vi "Bertta_v06_2.vi"() -> ()   [LabVIEW 2015]
uses:
  x64/Debug/BERTTA.dll
panel:
  in  "s":bool
  out "Numeric 4":dbl
  in  "Tab Control":T1(tab)
  in  "Description":string
  in  "Project name":string
  in  "User (initials)":string
  out "Tr":dbl
  out "Tj":dbl
  out "Numeric 2":dbl
  out "Numeric 3":dbl
  out "Numeric":dbl
  out "Mettler 5":dynamicdata(graph)
  out "Temp":dynamicdata(graph)
  out "Mettler":dynamicdata(graph)
  in  "Balances":bool[](array[boolean])
  out "Waveform Chart 3":dynamicdata(graph)
  out "Table":string[][](table)
  in  "Headers":string[](array[string])
  in  "?":bool
  in  "Seq":dbl[][](array[numeric])=[[20.0, 40.0, 50.0], [40.0, 50.0, 20.0], [3.0, 3.0, 3.0]]
  out "Sp":dbl
  out "T":dbl
  out "Tinit":dbl
  out "Tset":dbl
  out "Time limit":dbl
  out "Step":i32
  out "Waveform Chart":dynamicdata(graph)
  in  "Tbypass":dbl=20.0
  in  "Tfail":dbl=22.0
  in  "err":i32
  in  "PAUSE":bool
  out "Tj in":dbl
  out "Tj out":dbl
  out "DT":dbl
  out "Elapsed":i32 format="%<%H:%M:%S>t"
  out "Waveform Chart 2":dynamicdata(graph)
  out "Rate (g/s)":dbl
  out "Time (s)":dbl
  out "Target (g)":dbl
  in  "Seq 2":dbl[][](array[numeric])=[[20.0, 60.0, 40.0], [60.0, 40.0, 20.0], [100.0, 100.0, 100.0]]
  out "Weight (1)":dbl
  out "target reached":i32
  out "x/y":dbl
  out "bal_previous":i32
  out "Step":i32
  in  "?":bool
  in  "Bypass ramp":dbl
  in  "bypass 2":bool
  out "DAQ assistant (4-20 mA)":dbl
  out "Step":i32
  out "bal_previous":i32
  out "x/y":dbl
  out "target reached":i32
  out "Waveform Chart 5":dynamicdata(graph)
  out "Weight (2)":dbl
  out "Rate (g/s)":dbl
  out "Time (s)":dbl
  out "Target (g)":dbl
  in  "Seq 3":dbl[][](array[numeric])=[[20.0, 60.0, 40.0], [60.0, 40.0, 20.0], [100.0, 100.0, 100.0]]
  in  "Boolean":bool
  in  "Bypass ramp":dbl
  in  "bypass":bool
  out "RS232 to Ismatec":dbl
  in  "Boolean 2":bool
  out "Step":i32
  out "bal_previous":i32
  out "x/y":dbl
  out "target reached":i32
  out "Waveform Chart 6":dynamicdata(graph)
  out "Weight (3)":dbl
  out "Rate (g/s)":dbl
  out "Time (s)":dbl
  out "Target (g)":dbl
  in  "Seq 4":dbl[][](array[numeric])=[[20.0, 60.0, 40.0], [60.0, 40.0, 20.0], [100.0, 100.0, 100.0]]
  in  "Boolean 3":bool
  out "Step":i32
  out "bal_previous":i32
  out "x/y":dbl
  out "target reached":i32
  out "Waveform Chart 7":dynamicdata(graph)
  out "Weight (4)":dbl
  out "Rate (g/s)":dbl
  out "Time (s)":dbl
  out "Target (g)":dbl
  in  "Seq 5":dbl[][](array[numeric])=[[20.0, 60.0, 40.0], [60.0, 40.0, 20.0], [100.0, 100.0, 100.0]]
  out "RPM":dbl
  out "Torque":dbl
  in  "Set RPM":dbl(slide) scale=0.0..500.0
  out "Waveform Chart 4":dynamicdata(graph)
  in  "?":T2(tab)
  in  "Device port":dbl=9.0
  out "Debug msg":dbl
  in  "Device port":dbl=13.0
  in  "Device port":i32=10
  in  "Device port 2":i32=11
  in  "Device port 3":i32=12
  in  "Device port 4":i32=15
  # "1"
  # "2"
  # "3"
  # "4"
  # "Step 1"
  # "Step 2"
  # "Step 3"
  # "Step 4"
  # "Step 1"
  # "Step 2"
  # "Step 3"
  # "Step 4"
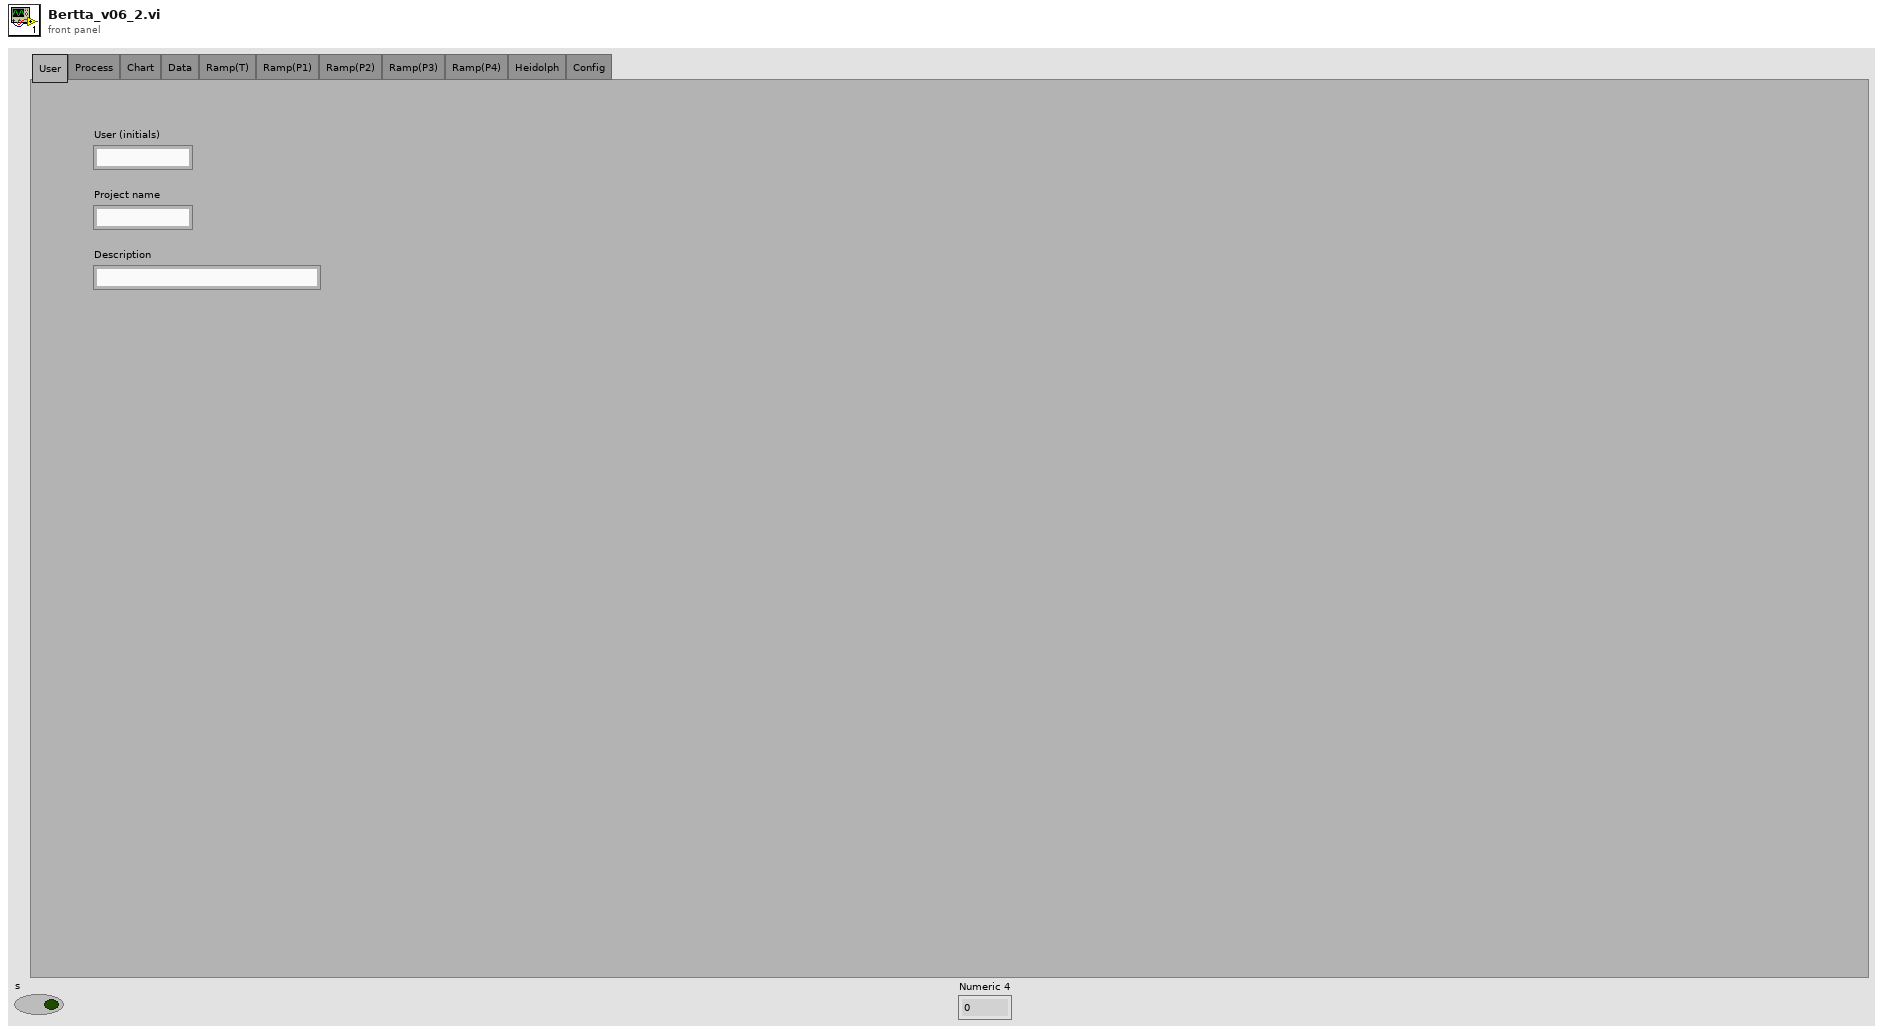
[diagram p1: front panel]
types:
  T1 = enum32{"User", "Process", "Chart", "Data", "Ramp(T)", "Ramp(P1)", "Ramp(P2)", "Ramp(P3)", "Ramp(P4)", "Heidolph", "Config"}
  T2 = enum32{"DB / File", "Lauda", "Heidolph", "Mettler 1", "Mettler 2", "Mettler 3", "Ismatec 1"}
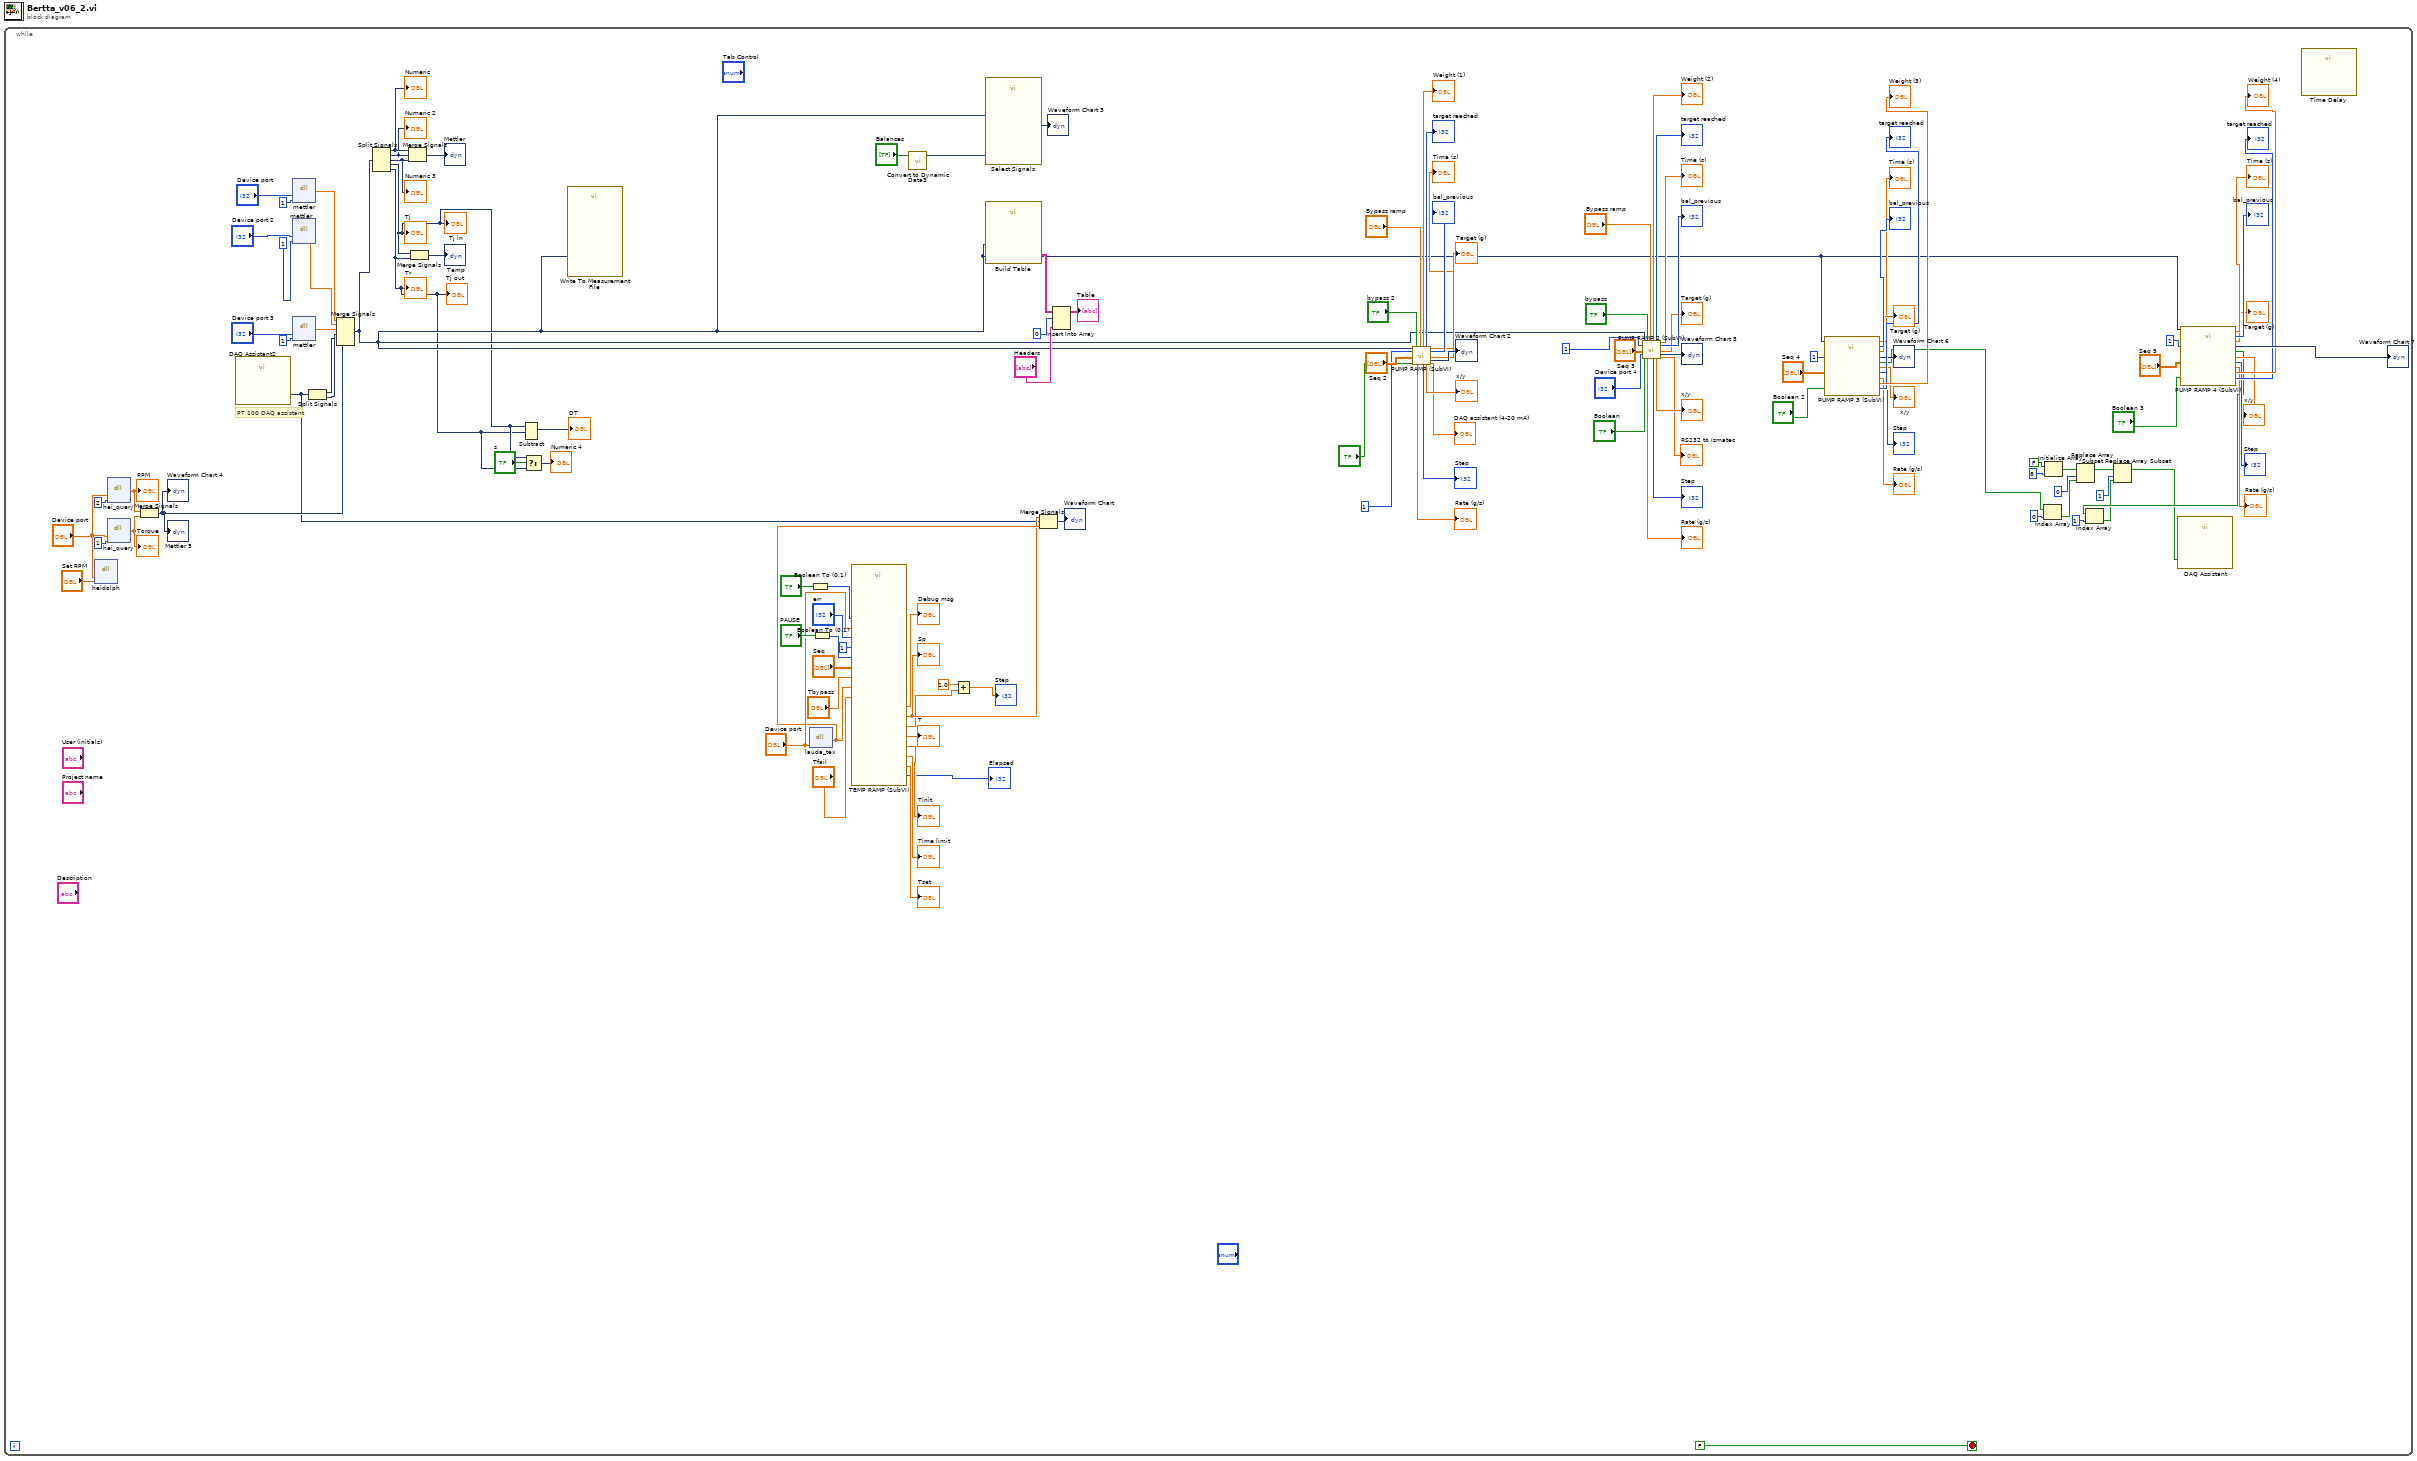
[diagram p0: block diagram]
diagram:
  n1 = while {
    stop <- FALSE stop-if-true
    # "PT 100 DAQ assistant"
    n2 = dll-call lib="C:/Users/shresplab/OneDrive - Kemira Oyj/Documents/Visual Studio 2017/Projects/Bertta/BERTTA/x64/Debug/BERTTA.dll" fn="heidolph"("port"="Device port", "speed"="Set RPM") -> ()  [unwired: 6 in, 2 out]
    n3 = dll-call lib="C:/Users/shresplab/OneDrive - Kemira Oyj/Documents/Visual Studio 2017/Projects/Bertta/BERTTA/x64/Debug/BERTTA.dll" fn="hei_query"("port"="Device port", "q"=2) -> ("return type"=w113:dbl)  [unwired: 5 in, 2 out]
    "RPM" <- w113
    n4 = dll-call lib="C:/Users/shresplab/OneDrive - Kemira Oyj/Documents/Visual Studio 2017/Projects/Bertta/BERTTA/x64/Debug/BERTTA.dll" fn="hei_query"("port"="Device port", "q"=1) -> ("return type"=w112:dbl)  [unwired: 5 in, 2 out]
    "Torque" <- w112
    n5 = Merge Signals(w113, w112) -> (w19:dynamicdata)
    "Waveform Chart 4" <- w19
    "Mettler 5" <- w19
    n6 = call "DAQ Assistant2"() -> ("data"=w4:dynamicdata)  [unwired: 17 in, 2 out]
    n7 = dll-call lib="C:/Users/shresplab/OneDrive - Kemira Oyj/Documents/Visual Studio 2017/Projects/Bertta/BERTTA/x64/Debug/BERTTA.dll" fn="mettler"("port"="Device port", "msg"=1) -> ("return type"=w85:dbl)  [unwired: 5 in, 2 out]
    n8 = dll-call lib="C:/Users/shresplab/OneDrive - Kemira Oyj/Documents/Visual Studio 2017/Projects/Bertta/BERTTA/x64/Debug/BERTTA.dll" fn="mettler"("port"="Device port 2", "msg"=1) -> ("return type"=w84:dbl)  [unwired: 5 in, 2 out]
    n9 = dll-call lib="C:/Users/shresplab/OneDrive - Kemira Oyj/Documents/Visual Studio 2017/Projects/Bertta/BERTTA/x64/Debug/BERTTA.dll" fn="mettler"("port"="Device port 3", "msg"=1) -> ("return type"=w71:dbl)  [unwired: 5 in, 2 out]
    n10 = Split Signals(w4) -> (w10:dynamicdata, w51:dynamicdata)  [unwired: 2 in]
    n11 = Merge Signals(w85, w84, w71, w51, w10, w19) -> (w17:dynamicdata)
    n12 = Split Signals(w17) -> (w24:dynamicdata, w22:dynamicdata, w21:dynamicdata, w16:dynamicdata, w15:dynamicdata)  [unwired: 5 in]
    "Numeric" <- w24
    "Numeric 2" <- w22
    "Numeric 3" <- w21
    "Tr" <- w15
    "Tj" <- w16
    "Tj in" <- w16
    "Tj out" <- w15
    n13 = Merge Signals(w24, w22, w21) -> (→"Mettler":dynamicdata)
    n14 = Merge Signals(w16, w15) -> (→"Temp":dynamicdata)
    n15 = Subtract(1:w15, 2:w16) -> (0:→"DT":dynamicdata)  [unwired: 1 in, 1 out]
    n16 = Select(t=w16, s="s", f=w15) -> (s? t:f=→"Numeric 4":dynamicdata)
    n17 = call "Write To Measurement File"("Signals"=w17) -> ()  [unwired: 16 in, 3 out]
    n18 = dll-call lib="C:/Users/shresplab/OneDrive - Kemira Oyj/Documents/Visual Studio 2017/Projects/Bertta/BERTTA/x64/Debug/BERTTA.dll" fn="lauda_tex"("port"="Device port") -> ("return type"=w11:dbl)  [unwired: 4 in, 2 out]
    n19 = Boolean To (0,1)(Boolean="?") -> (0, 1=w66:i16)
    n20 = Boolean To (0,1)(Boolean="PAUSE") -> (0, 1=w20:i16)
    n21 = call "TEMP RAMP (SubVI).vi"("Device port"="Device port", "enable"=i16 1 ("Numeric"), "Tbyp"="Tbypass", "pause"=w20, "Seq"="Seq", "Tcurrent"=w11, "bypass"=w66, "err"="err", "Tfail"="Tfail") -> ("Step out"=w3:dbl, "T"=→"T":dbl, "Sp"=w7:dbl, "elapsed"=→"Elapsed":i32, "tr"=→"Time limit":dbl, "Debug msg"=→"Debug msg":dbl, "Tset"=→"Tset":dbl, "Tinit"=→"Tinit":dbl)  [unwired: 3 in]
    "Sp" <- w7
    n22 = call "Convert to Dynamic Data3"("Array"="Balances") -> ("Dynamic Data Type"=w119:dynamicdata)  [unwired: 3 in]
    n23 = Add(x=1.0, y=w3) -> (x+y=→"Step":dbl)
    n24 = call "Select Signals"("Selector Input"=w119, "Signals"=w17) -> ("Signal Out"=→"Waveform Chart 3":dynamicdata)  [unwired: 8 in, 1 out]
    n25 = call "Build Table"("Signals"=w17) -> ("Table"=w122:string[][])  [unwired: 4 in, 6 out]
    n26 = Merge Signals(w7, w4, w11) -> (→"Waveform Chart":dynamicdata)
    n27 = Insert Into Array(array=w122, index (row)=0, new element="Headers") -> (→"Table":string[][])  [unwired: 1 in]
    n28 = call "PUMP RAMP (SubVI).vi"("Dynamic Data"=w17, "Numeric"=i16 1, "Seq in"="Seq 2", 5:"?", "bypass"="bypass 2", "bypass RPM"="Bypass ramp") -> ("Rate (g/s)"=→"Rate (g/s)":dbl, "Weight (S1)"=→"Weight (1)":dbl, "Step 2"=→"Step":i32, "target reached"=→"target reached":i32, "x/y"=→"x/y":dbl, "Time (s)"=→"Time (s)":dbl, "bal_previous"=→"bal_previous":i32, "Target (g)"=→"Target (g)":dbl, "Waveform Chart 2"=→"Waveform Chart 2":dynamicdata, "DAQ assistant (4-20 mA)"=→"DAQ assistant (4-20 mA)":dbl)  [unwired: 4 in]
    n29 = call "PUMP RAMP 2 (SubVI).vi"("Dynamic Data"=w17, "Numeric"=i16 1, "Seq in"="Seq 3", "Device port"="Device port 4", "enable"="Boolean", "bypass"="bypass", "bypass RPM"="Bypass ramp") -> ("Rate (g/s)"=→"Rate (g/s)":dbl, "Weight (S1)"=→"Weight (2)":dbl, "Step 2"=→"Step":i32, "target reached"=→"target reached":i32, "x/y"=→"x/y":dbl, "Time (s)"=→"Time (s)":dbl, "bal_previous"=→"bal_previous":i32, "Target (g)"=→"Target (g)":dbl, "Waveform Chart 2"=→"Waveform Chart 5":dynamicdata, "RS232 to Ismatec"=→"RS232 to Ismatec":dbl)  [unwired: 3 in]
    n30 = call "PUMP RAMP 3 (SubVI).vi"("Dynamic Data"=w17, "Numeric"=i16 1, "Seq in"="Seq 4", "Boolean"="Boolean 2") -> ("Weight (S1)"=→"Weight (3)":dbl, "target reached"=→"target reached":i32, "Time (s)"=→"Time (s)":dbl, "bal_previous"=→"bal_previous":i32, "Target (g)"=→"Target (g)":dbl, "Waveform Chart 2"=→"Waveform Chart 6":dynamicdata, "Rate (g/s)"=→"Rate (g/s)":dbl, "Step 2"=→"Step":i32, "x/y"=→"x/y":dbl, "DAQ assistant (PAM i/o)"=w36:bool[])  [unwired: 2 in]
    n31 = Index Array(array=w36, index=0) -> (element=w30:bool)
    n32 = Initialize Array(FALSE ("element"), 8 ("dimension size")) -> (w32:bool[])
    n33 = Replace Array Subset(array=w32, new element=w30, index=0) -> (w26:bool[])
    n34 = call "PUMP RAMP 4 (SubVI).vi"("Dynamic Data"=w17, "Numeric"=i16 1, "Seq in"="Seq 5", "Boolean"="Boolean 3") -> ("Weight (S1)"=→"Weight (4)":dbl, "target reached"=→"target reached":i32, "Time (s)"=→"Time (s)":dbl, "bal_previous"=→"bal_previous":i32, "Target (g)"=→"Target (g)":dbl, "Waveform Chart 2"=→"Waveform Chart 7":dynamicdata, "Rate (g/s)"=→"Rate (g/s)":dbl, "Step 2"=→"Step":i32, "x/y"=→"x/y":dbl, "DAQ assistant (PAM i/o)"=w33:bool[])  [unwired: 2 in]
    n35 = Index Array(array=w33, index=1) -> (element=w28:bool)
    n36 = Replace Array Subset(array=w26, new element=w28, index=1) -> (w29:bool[])
    n37 = call "DAQ Assistant"("data"=w29) -> ()  [unwired: 17 in, 2 out]
    n38 = call "Time Delay"() -> ()  [unwired: 11 in, 1 out]
  }
